vi "SerialComMain.vi"() -> ()   [LabVIEW 2014]
uses:
  MainDataTypedef.ctl
  <vilib>/Instr/_visa.llb/VISA Configure Serial Port (Instr).vi
panel:
  out "bytes read":u32
  out "NowTime":timestamp
  in  "ClosePort":bool
  in  "OpenProt":bool
  in  "flow control":u16(ring) items=["None"=0, "XON/XOFF"=1, "RTS/CTS"=2, "DTR/DSR"=4]
  in  "stop bits":u16(ring)=10 items=["1.0"=10, "1.5"=15, "2.0"=20]
  in  "parity":u16(ring) items=["None", "Odd", "Even", "Mark", "Space"]
  in  "data bits":u16=8 min=5 max=8 step=1
  in  "baud rate":u32=9600
  in  "delay before read (ms)":u32=500
  in  "VISA resource name":refnum<visa-resource-name>="COM1"
  out "Response":string
  in  "Command":string="*IDN?\n"
  in  "SerialSend":bool
  out "MsgString":string
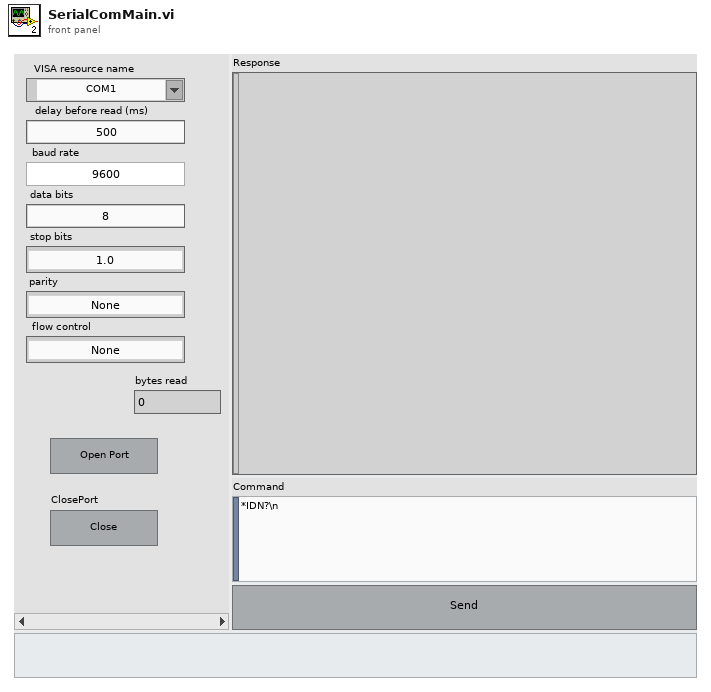
[diagram p1: front panel]
types:
  T1 = typedef "MainDataTypedef.ctl" = cluster{"NowTime":timestamp, "MsgString":string, "VISAResource":refnum<visa-resource-name>, "BytesRead":u32, "Respones":string, "PortOpen?":bool}
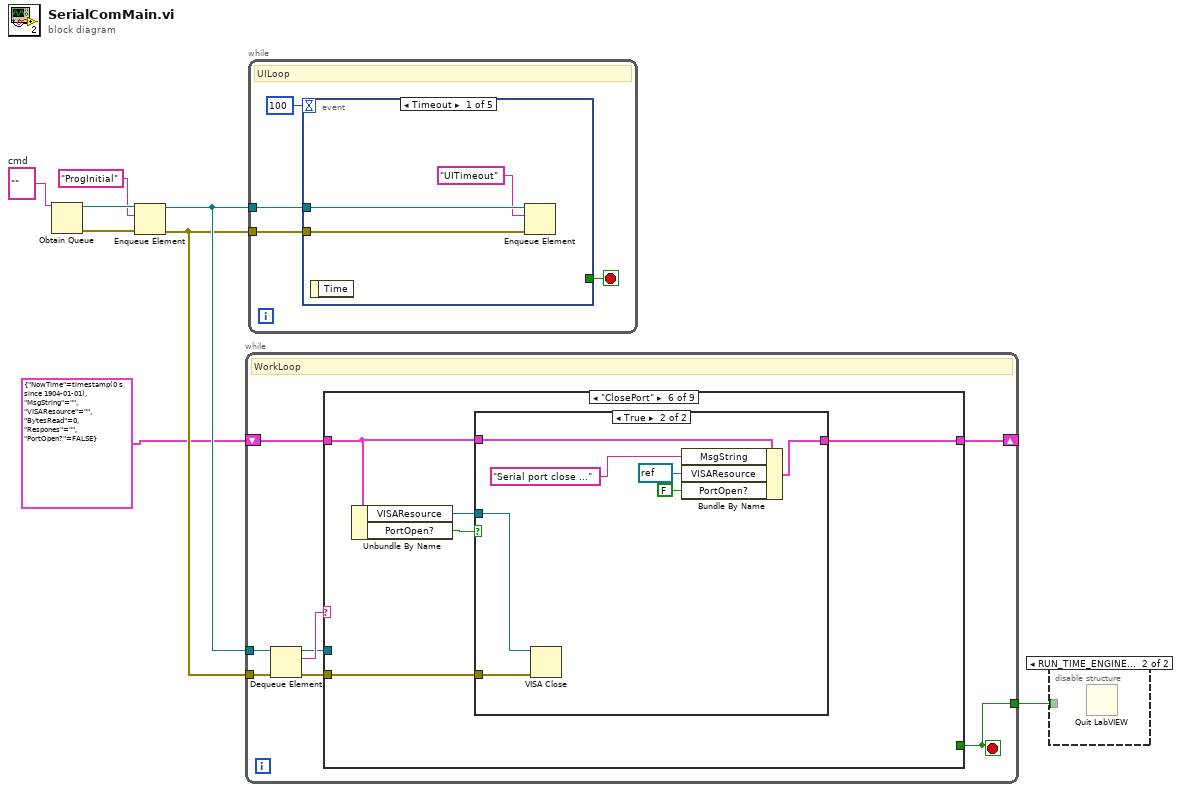
[diagram p0: block diagram]
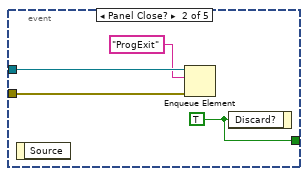
[diagram p3: hidden frame]
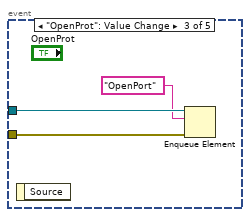
[diagram p4: hidden frame]
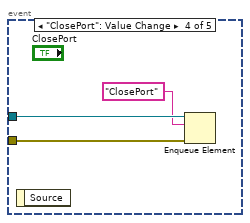
[diagram p5: hidden frame]
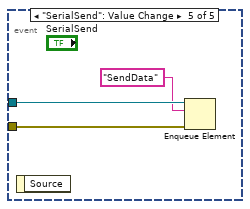
[diagram p6: hidden frame]
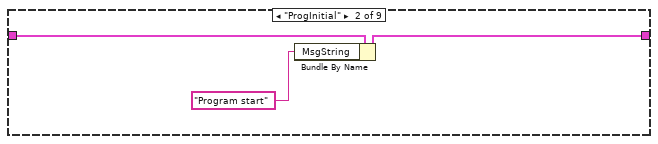
[diagram p8: hidden frame]
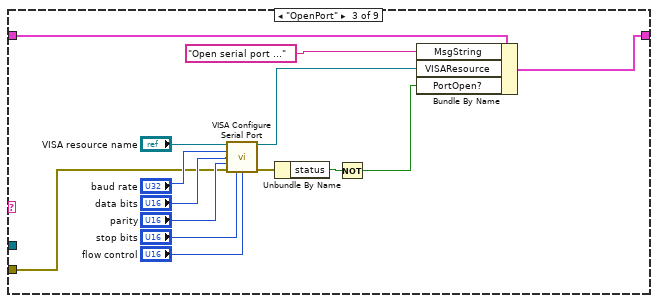
[diagram p9: hidden frame]
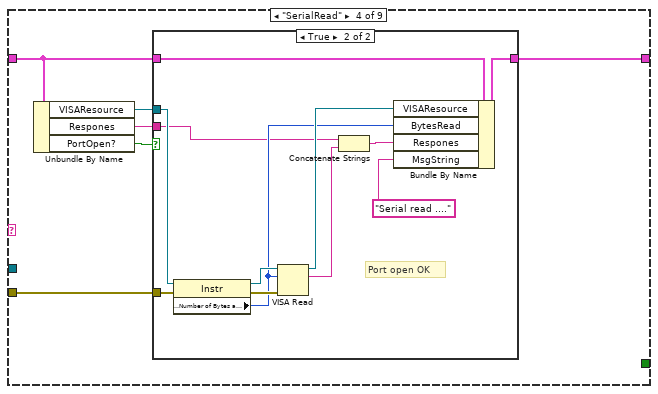
[diagram p10: hidden frame]
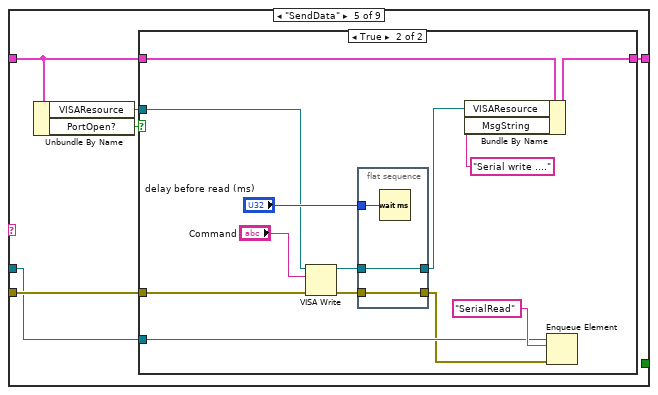
[diagram p12: hidden frame]
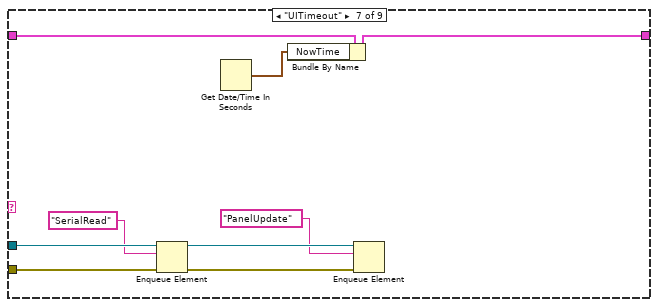
[diagram p15: hidden frame]
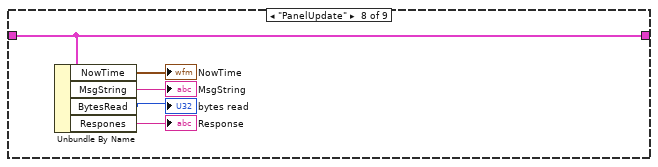
[diagram p16: hidden frame]
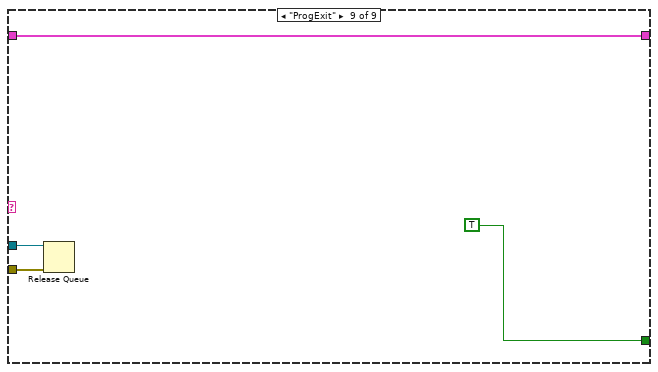
[diagram p17: hidden frame]
diagram:
  w6 = ""  # cmd
  n1 = Obtain Queue(element data type=w6) -> (queue out=w8:refnum<queue>, error out=w7:errorcluster)  [unwired: 4 in, 1 out]
  n2 = Enqueue Element(queue=w8, element="ProgInitial", error in (no error)=w7) -> (queue out=w4:refnum<queue>, error out=w3:errorcluster)  [unwired: 1 in, 1 out]
  n3 = while {
    tunnel: w4 -> [w16]
    tunnel: w3 -> [w15]
    shift-right: [w13] -> _
    shift-left: T1 {"NowTime"=timestamp(0 s since 1904-01-01), "MsgString"="", "VISAResource"="", "BytesRead"=0, "Respones"="", "PortOpen?"=FALSE} -> [w12]
    tunnel: [w9] -> w1
    stop <- w9 stop-if-true
    # "WorkLoop"
    n4 = Dequeue Element(queue=w16, error in (no error)=w15) -> (queue out=w11:refnum<queue>, element=w14:string, error out=w10:errorcluster)  [unwired: 1 in, 1 out]
    n5 = case shown="\"ClosePort\"" w14 {
      tunnel: [w17 w19 w33 w37 w56 w81 w97 w103 w107] -> w13
      tunnel: w12 -> [w17 w20 w34 w40 w59 w80 w98 w103 w107]
      tunnel: w11 -> [_ _ _ _ w54 _ w95 _ w106]
      tunnel: w10 -> [_ _ w25 w38 w57 w78 w94 _ w105]
      tunnel: [_ _ _ _ _ _ _ _ TRUE ("Discard?")] -> w9
      frame Default {
      }
      frame "ProgInitial" {
        n6 = Bundle By Name(cluster=w20, "MsgString"="Program start" ("message")) -> (w19:T1)
      }
      frame "OpenPort" {
        n7 = call-poly "VISA Configure Serial Port"("VISA resource name"="VISA resource name", "baud rate (9600)"="baud rate", "data bits (8)"="data bits", "parity (0:none)"="parity", "error in (no error)"=w25, "stop bits (10: 1 bit)"="stop bits", "flow control (0:none)"="flow control") -> ("VISA resource name out"=w24:refnum<visa-resource-name>, "error out"=w23:errorcluster)  [unwired: 2 in, 5 out]
        n8 = Unbundle By Name(w23) -> ("status"=w22:bool)
        n9 = Not(x=w22) -> (.not. x?=w21:bool)
        n10 = Bundle By Name(cluster=w34, "MsgString"="Open serial port ..." ("message"), "VISAResource"=w24, "PortOpen?"=w21) -> (w33:T1)
      }
      frame "SerialRead" {
        n11 = Unbundle By Name(w40) -> ("VISAResource"=w39:refnum<visa-resource-name>, "Respones"=w36:string, "PortOpen?"=w35:bool)
        n12 = case shown="True" w35 {
          tunnel: w40 -> [w41 w51]
          tunnel: w39 -> [_ w50]
          tunnel: w38 -> [_ w49]
          tunnel: [w41 w48] -> w37
          tunnel: w36 -> [_ w43]
          frame False {
            # "Port not open"
          }
          frame True {
            # "Port open OK"
            n13 = property class="Instr"(reference=w50, error in=w49) -> (reference out=w52:refnum<visa-resource-name>, error out=w53:errorcluster, "Serial Settings:Number of Bytes at Serial Port"=w46:u32)
            n14 = VISA Read(VISA resource name=w52, byte count=w46, error in (no error)=w53) -> (VISA resource name out=w47:refnum<visa-resource-name>, read buffer=w45:string)  [unwired: 2 out]
            n15 = Concatenate Strings(w43, w45) -> (w44:string)
            n16 = Bundle By Name(cluster=w51, "VISAResource"=w47, "BytesRead"=w46, "Respones"=w44, "MsgString"="Serial read ....") -> (w48:T1)
          }
        }
      }
      frame "SendData" {
        n17 = Unbundle By Name(w59) -> ("VISAResource"=w58:refnum<visa-resource-name>, "PortOpen?"=w55:bool)
        n18 = case shown="True" w55 {
          tunnel: w59 -> [w60 w73]
          tunnel: w58 -> [_ w66]
          tunnel: w57 -> [_ w64]
          tunnel: [w60 w72] -> w56
          tunnel: w54 -> [_ w62]
          frame False {
            # "Port not open"
          }
          frame True {
            n19 = VISA Write(VISA resource name=w66, write buffer="Command", error in (no error)=w64) -> (VISA resource name out=w68:refnum<visa-resource-name>, error out=w67:errorcluster)  [unwired: 1 out]
            n20 = flat-sequence {
              tunnel: w67 -> [w75]
              tunnel: [w75] -> w61
              tunnel: w68 -> [w74]
              tunnel: [w74] -> w65
              tunnel: "delay before read (ms)" -> [w76]
              frame #0 {
                n21 = Wait (ms)(milliseconds to wait=w76) -> ()  [unwired: 1 out]
              }
            }
            n22 = Bundle By Name(cluster=w73, "VISAResource"=w65, "MsgString"="Serial write ....") -> (w72:T1)
            n23 = Enqueue Element(queue=w62, element="SerialRead", error in (no error)=w61) -> ()  [unwired: 1 in, 3 out]
          }
        }
      }
      frame "ClosePort" {
        n24 = Unbundle By Name(w80) -> ("VISAResource"=w79:refnum<visa-resource-name>, "PortOpen?"=w77:bool)
        n25 = case shown="True" w77 {
          tunnel: [w82 w89] -> w81
          tunnel: w80 -> [w82 w87]
          tunnel: w79 -> [_ w86]
          tunnel: w78 -> [_ w85]
          frame False {
            # "port not open"
          }
          frame True {
            n26 = VISA Close(VISA resource name=w86, error in (no error)=w85) -> ()  [unwired: 1 out]
            n27 = Bundle By Name(cluster=w87, "MsgString"="Serial port close ..." ("message"), "VISAResource"=refnum<visa-resource-name> refnum, "PortOpen?"=FALSE) -> (w89:T1)
          }
        }
      }
      frame "UITimeout" {
        n28 = Enqueue Element(queue=w95, element="SerialRead", error in (no error)=w94) -> (queue out=w93:refnum<queue>, error out=w92:errorcluster)  [unwired: 1 in, 1 out]
        n29 = Get Date/Time In Seconds() -> (seconds since 1Jan1904=w96:timestamp)
        n30 = Bundle By Name(cluster=w98, "NowTime"=w96) -> (w97:T1)
        n31 = Enqueue Element(queue=w93, element="PanelUpdate", error in (no error)=w92) -> ()  [unwired: 1 in, 3 out]
      }
      frame "PanelUpdate" {
        n32 = Unbundle By Name(w103) -> ("NowTime"=→"NowTime":timestamp, "MsgString"=→"MsgString":string, "BytesRead"=→"bytes read":u32, "Respones"=→"Response":string)
      }
      frame "ProgExit" {
        n33 = Release Queue(queue=w106, error in (no error)=w105) -> ()  [unwired: 1 in, 3 out]
      }
    }
  }
  n34 = while {
    tunnel: w4 -> [w110]
    tunnel: w3 -> [w109]
    stop <- w108 stop-if-true
    # "UILoop"
    n35 = event shown="[0] Timeout" {
      selector: _ -> [_ _ _ _ _]
      dyn-events: _ -> [_ _ _ _ _]
      timeout: 100 -> [_ _ _ _ _]
      tunnel: w110 -> [w114 w118 w121 w124 w127]
      tunnel: w109 -> [w113 w117 w120 w123 w126]
      tunnel: [_ w116 _ _ _] -> w108
      event Timeout {
        n36 = event-data() -> ()  [unwired: 1 in, 1 out]
        n37 = Enqueue Element(queue=w114, element="UITimeout", error in (no error)=w113) -> ()  [unwired: 1 in, 3 out]
      }
      event Panel Close? {
        w116 = TRUE ("Discard?")
        n38 = event-data() -> ()  [unwired: 1 in, 1 out]
        n39 = Enqueue Element(queue=w118, element="ProgExit", error in (no error)=w117) -> ()  [unwired: 1 in, 3 out]
        n40 = event-data("Discard?"=w116) -> ()  [unwired: 1 in, 1 out]
      }
      event "OpenProt": Value Change {
        n41 = event-data() -> ()  [unwired: 1 in, 1 out]
        n42 = Enqueue Element(queue=w121, element="OpenPort", error in (no error)=w120) -> ()  [unwired: 1 in, 3 out]
      }
      event "ClosePort": Value Change {
        n43 = event-data() -> ()  [unwired: 1 in, 1 out]
        n44 = Enqueue Element(queue=w124, element="ClosePort", error in (no error)=w123) -> ()  [unwired: 1 in, 3 out]
      }
      event "SerialSend": Value Change {
        n45 = event-data() -> ()  [unwired: 1 in, 1 out]
        n46 = Enqueue Element(queue=w127, element="SendData", error in (no error)=w126) -> ()  [unwired: 1 in, 3 out]
      }
    }
  }
  n47 = disable-structure shown="RUN_TIME_ENGINE==True" {
    disable-tunnel: w1 -> [_ _]
    frame condition #0 (active) {
    }
    frame condition #1 {
      n48 = Quit LabVIEW() -> ()  [unwired: 1 in]
    }
  }
